vi "factoriel.vi"() -> ()   [LabVIEW 2020]
panel:
  out "resultat":dbl
  in  "factoriel":dbl
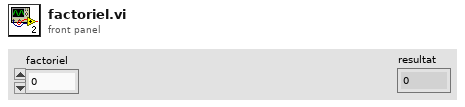
[diagram p1: front panel]
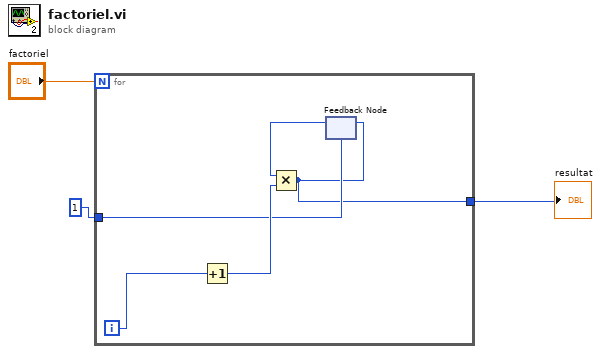
[diagram p0: block diagram]
diagram:
  n1 = for {
    N: "factoriel" -> [_]
    tunnel: [w4] -> w1
    tunnel: 1 -> [w5]
    i -> [w8]
    n2 = Increment(x=w8) -> (x+1=w7:i32)
    n3 = feedback #1(w5) -> (w6:i32)
    n4 = Multiply(x=w6, y=w7) -> (x*y=w4:i32)
    n5 = feedback-in #1(w4) -> ()
  }
  "resultat" <- w1
